vi "GradientThresholdProperty.vi"(7 "Write?":bool, 8 "error in (no error)":errorcluster, 10 "Value in":dbl, 11 "Barcode Detector in":refnum<class "Barcode Detector.lvclass">) -> (0 "error out":errorcluster, 3 "Value out":dbl)   [LabVIEW 2020, in "feature_detection.lvlib" / "Barcode Detector.lvclass"]
uses:
  Barcode Detector.lvclass
  Barcode Detector.lvclass/Barcode Detector.ctl
  common/common.lvlib
  common/bin/gartoolkit_fd_32-1.dll
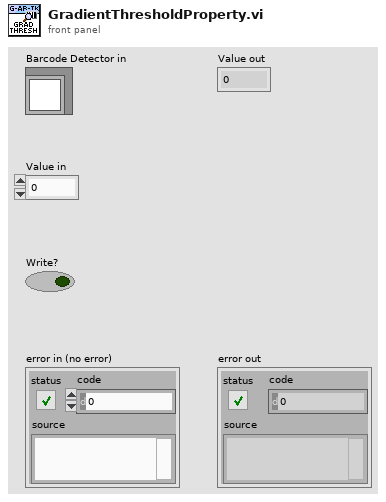
[diagram p1: front panel]
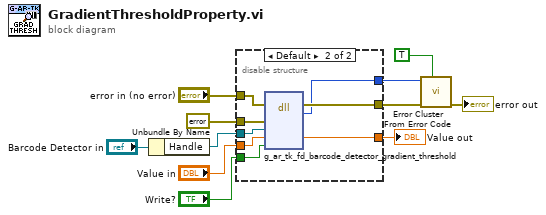
[diagram p0: block diagram]
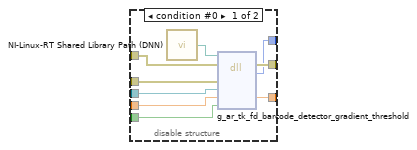
[diagram p2: hidden frame]
diagram:
  n1 = Unbundle By Name("Barcode Detector in") -> ("Handle"=w7:refnum<data-value>)
  n2 = disable-structure shown="Default" {
    disable-tunnel: "error in (no error)" -> [w20 w28]
    disable-tunnel: errorcluster {"status"=FALSE, "code"=0, "source"=""} ("error constant") -> [w19 w27]
    disable-tunnel: w7 -> [w18 w26]
    disable-tunnel: "Value in" -> [w17 w25]
    disable-tunnel: "Write?" -> [w16 w24]
    disable-tunnel: [w15 w23] -> w4
    disable-tunnel: [w14 w22] -> w3
    disable-tunnel: [w13 w21] -> w2
    frame condition #0 {
      n3 = call "NI-Linux-RT Shared Library Path (DNN).vi"() -> ("Path"=w12:path)
      n4 = dll-call lib="?" fn="g_ar_tk_fd_barcode_detector_gradient_threshold" ("g_ar_toolkit.*.*:g_ar_tk_capture_context_create")(path in=w12, error in=w20, "error_cluster"=w19, "Detector_EDVR"=w18, "Value"=w17, "Write"=w16) -> (error out=w15:errorcluster, "return type"=w14:i32, "Value"=w13:dbl)  [unwired: 4 in, 1 out]
    }
    frame condition #1 (active) {
      n5 = dll-call lib="C:/serenial/lib/g-augmented-reality-toolkit/LabVIEW/common/bin/gartoolkit_fd_*-1.*" fn="g_ar_tk_fd_barcode_detector_gradient_threshold" ("g_ar_toolkit.*.*:g_ar_tk_capture_context_create")(error in=w28, "error_cluster"=w27, "Detector_EDVR"=w26, "Value"=w25, "Write"=w24) -> (error out=w23:errorcluster, "return type"=w22:i32, "Value"=w21:dbl)  [unwired: 5 in, 1 out]
    }
  }
  "Value out" <- w2
  n6 = call <vilib>:"Error Cluster From Error Code.vi"("show call chain? (False)"=TRUE, "error in (no error)"=w4, "error code (0)"=w3) -> ("error out"=→"error out":errorcluster)  [unwired: 6 in]
